vi "DAC.vi"() -> ()   [LabVIEW 2010]
uses:
  <vilib>/eio/EIONode/EIONode.xnode
  <vilib>/Platform/TimedLoop/XDataNode/wakeup.ctl
  <vilib>/Platform/TimedLoop/XDataNode/XDNodeRunTimeDep.lvlib
  <vilib>/Platform/TimedLoop/XDataNode/nitl_modes.ctl
  <vilib>/Platform/TimedLoop/XDataNode/timing_clust.ctl
  <vilib>/Platform/TimedLoop/XDataNode/XDataNode.xnode
panel:
  in  "setBufferGainV_DD":bool
  in  "setLDACMode":bool
  in  "dataAndControlResetButton":bool
  in  "stop":bool
  in  "V_DD":enum16{"as reference", "not as reference"}(ring)
  in  "Gain":enum16{"Range 0...V_ref", "Range 0...2V_ref"}(ring)
  in  "Buffer mode":enum16{"unbuffered", "buffered"}(ring)
  out "loop counter":i32
  out "write counter":i32
  out "current bit":bool
  out "U16 data word":bool[](array[boolean])
  in  "dataResetButton":bool
  in  "Channel":u8 max=7 step=1
  in  "Voltage":u16 max=4095
  in  "startButton":bool
  in  "LDAC mode":T1(ring)
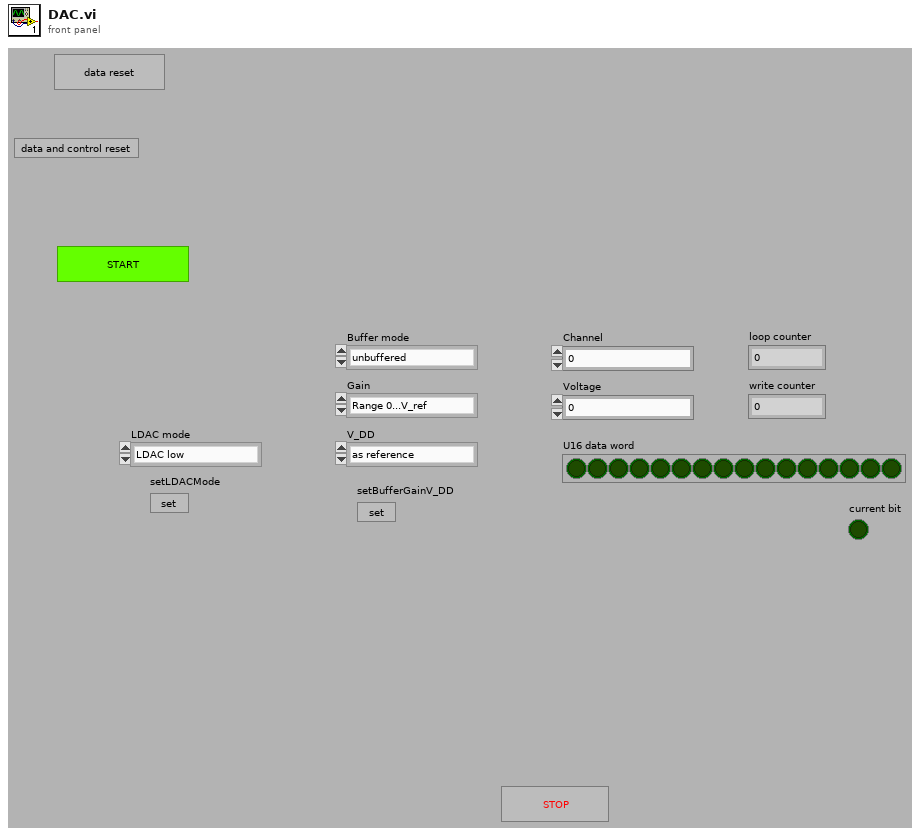
[diagram p1: front panel]
types:
  T1 = enum16{"LDAC low", "LDAC high", "LDAC single update"}
  T2 = typedef "XDNodeRunTimeDep.lvlib/timing_clust.ctl" = cluster{"Expected End [f-1]":u64, "Actual End [f-1]":u64, "Finished Late? [f-1]":bool, "Expected End [i-1]":u64, "Actual End [i-1]":u64, "Finished Late? [i-1]":bool, "Expected Start [i]":u64, "Actual Start [i]":u64, "Expected Start [f]":u64, "Actual Start [f]":u64, "Source Name":string, "Structure Name":string, "Period":i64, "Deadline":i64, "Offset":i64, "Start":i64, "Priority":i32, "Timeout":i32, "Mode":T3, "Wakeup Reason":T4, "Error":errorcluster, "Source Type":string, "Secondary Source Type":string, "Global End Time":u64, "Global Start Time":u64, "Frame Duration":u64, "Iteration Duration":u64, "Assigned CPU":i32, "I/O Scan Engine Mode":u32}
  T3 = typedef "XDNodeRunTimeDep.lvlib/nitl_modes.ctl" = enum32{"No Change", "Process missed periods, maintain original phase", "Discard missed periods, maintain original phase", "Process missed periods, ignore original phase", "Discard missed periods, ignore original phase"}
  T4 = typedef "XDNodeRunTimeDep.lvlib/wakeup.ctl" = enum32{"Normal", "Aborted", "Asynchronous wakeup", "Timing source error", "Timed loop error", "Timeout"}
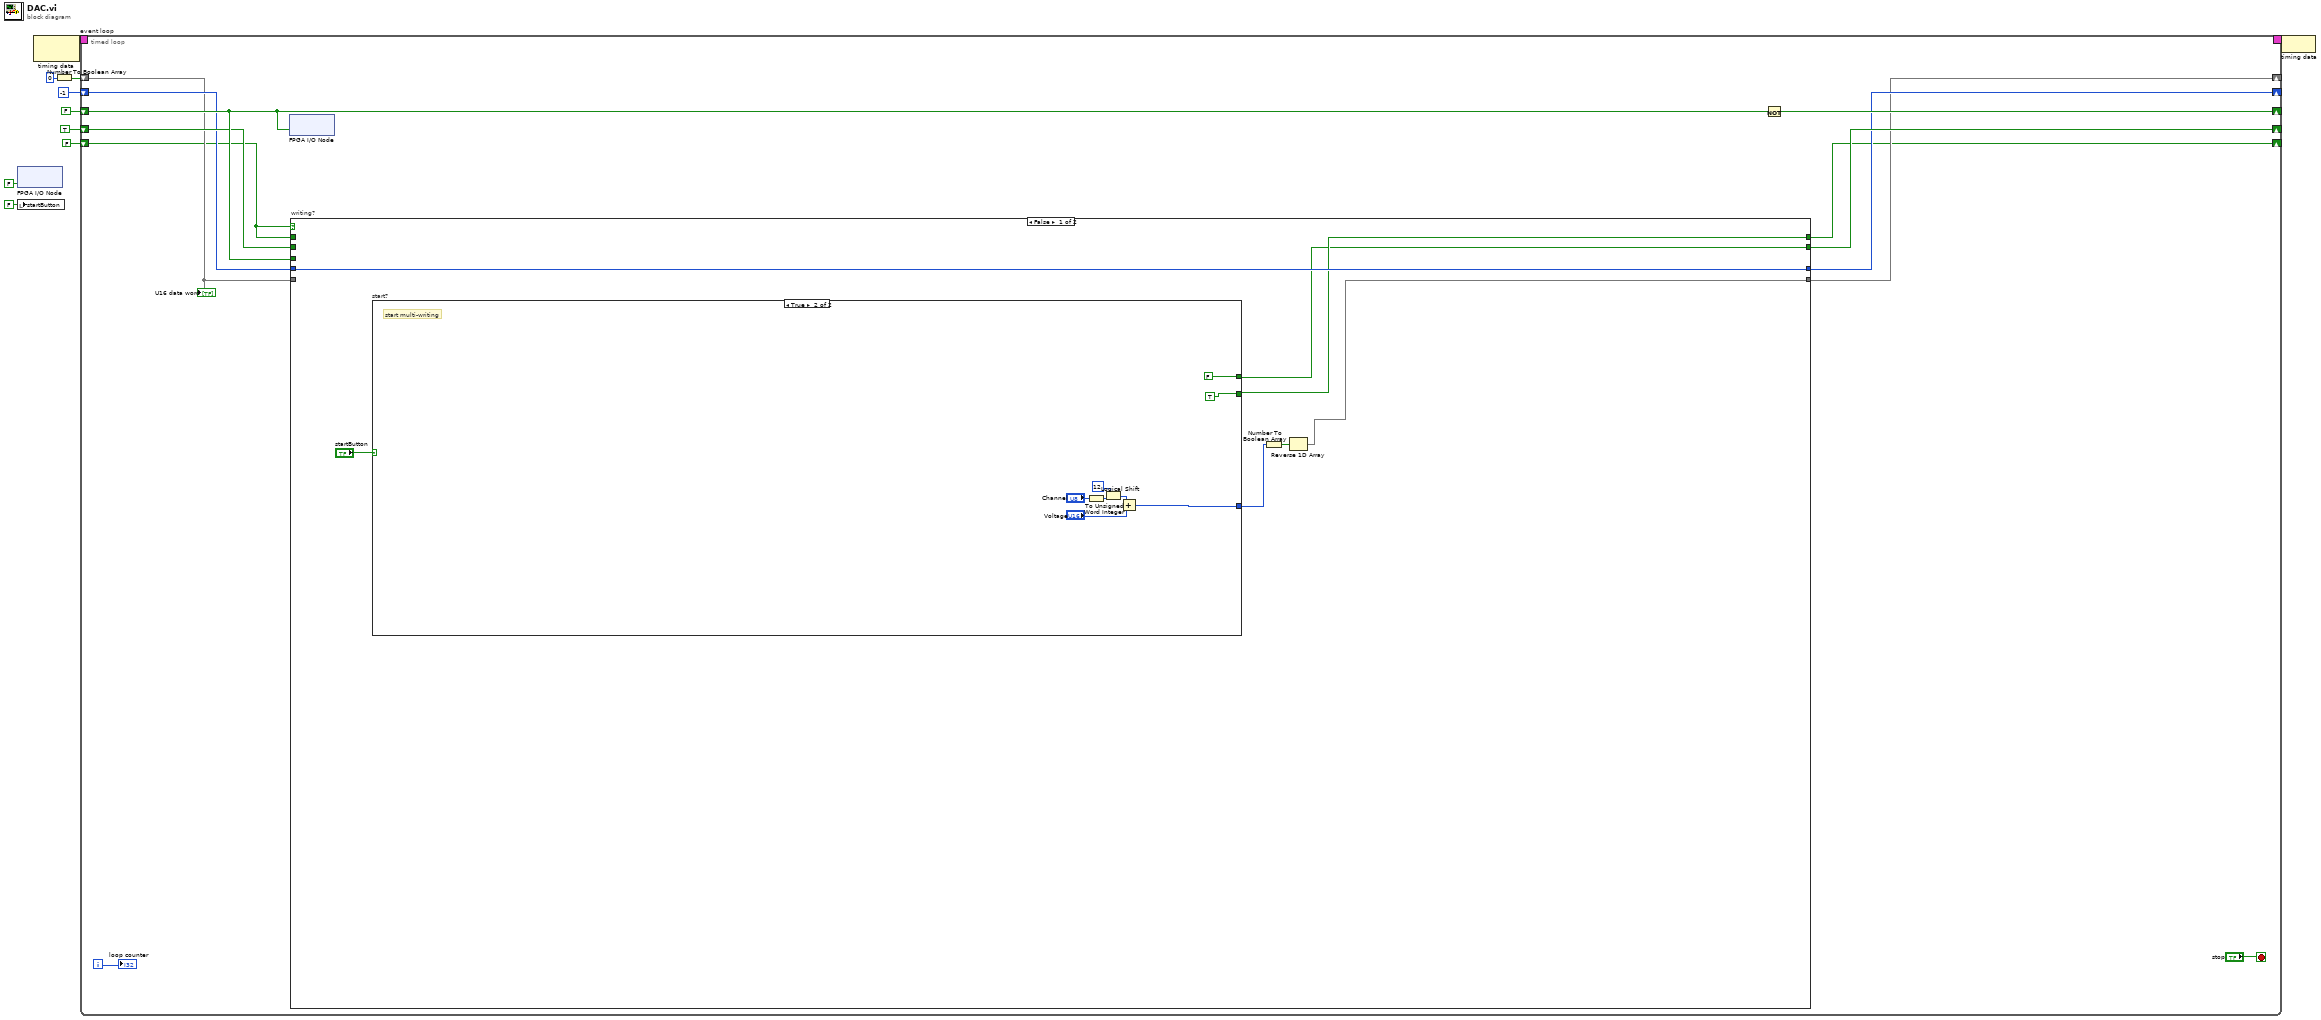
[diagram p0: block diagram]
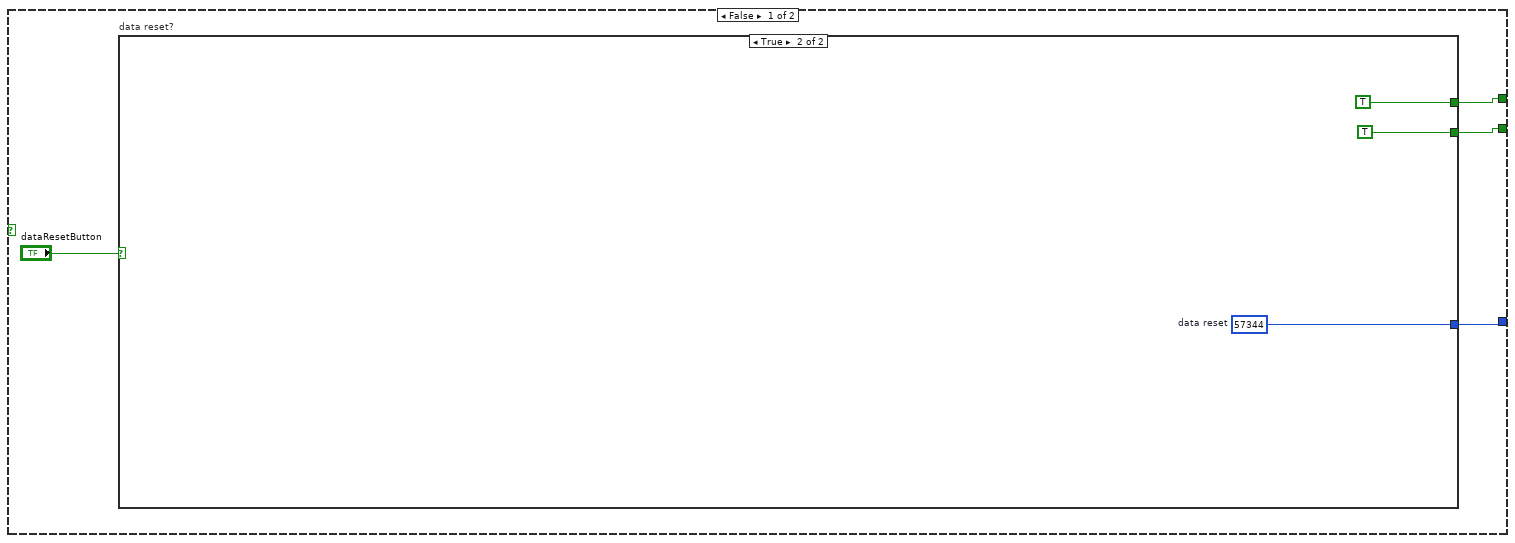
[diagram p2: hidden frame]
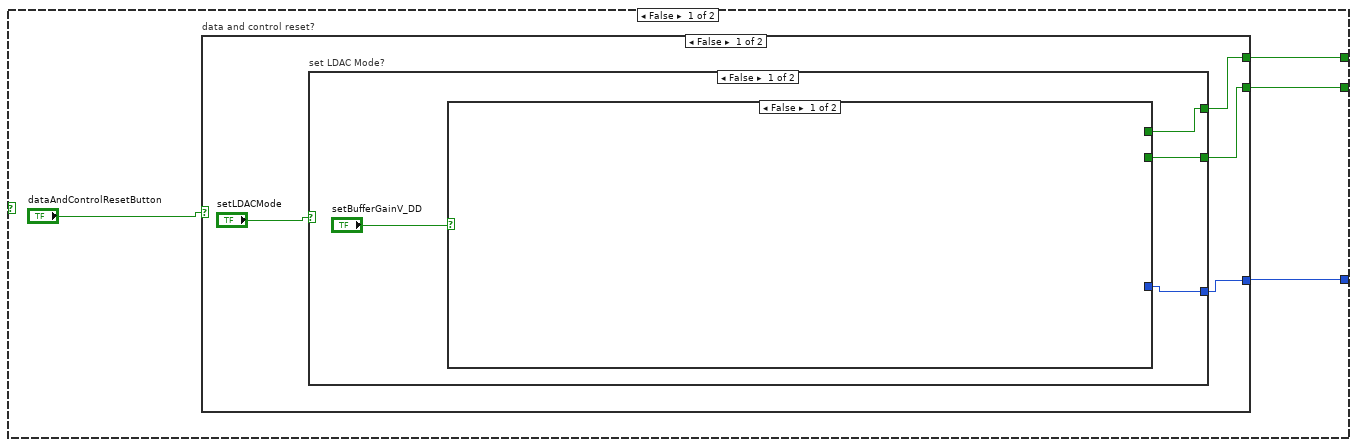
[diagram p3: hidden frame]
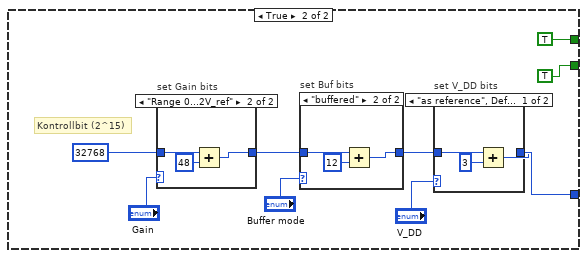
[diagram p4: hidden frame]
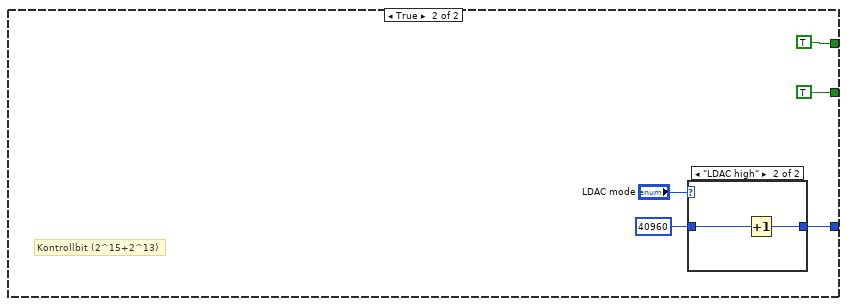
[diagram p8: hidden frame]
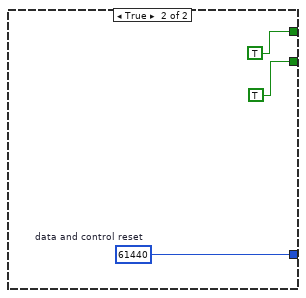
[diagram p10: hidden frame]
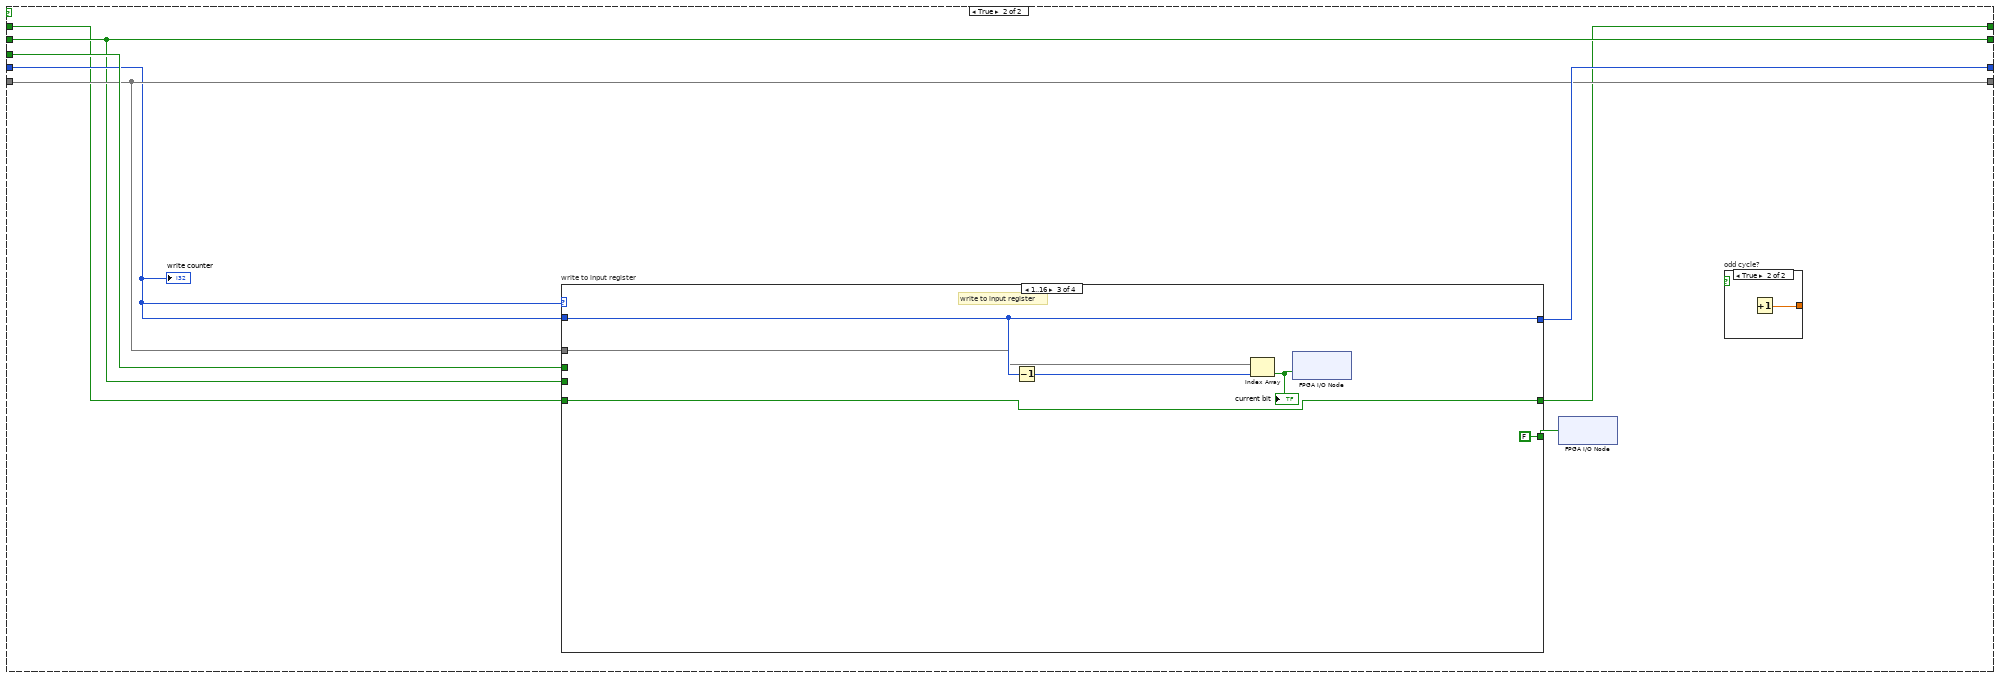
[diagram p11: hidden frame]
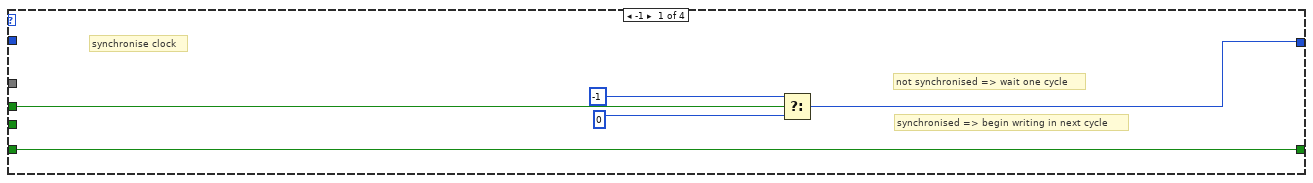
[diagram p12: hidden frame]
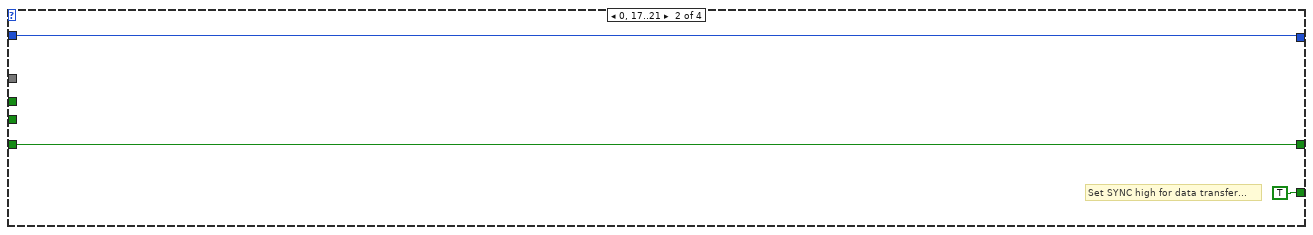
[diagram p13: hidden frame]
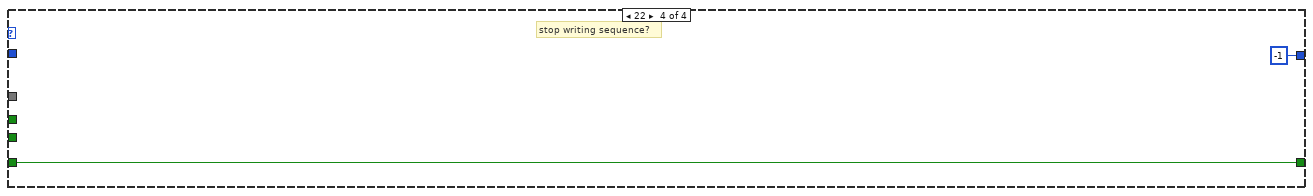
[diagram p14: hidden frame]
diagram:
  n1 = xnode "FPGA I/O Node"("LDAC"=FALSE) -> ()  [unwired: 1 in, 1 out]
  n2 = local write "startButton"(FALSE ("startButton")) -> ()
  n3 = node-c288() -> (w10:T2)  [unwired: 1 in]
  n4 = Number To Boolean Array(number=u16 0) -> (Boolean array=w4:bool[])
  n5 = timed-loop "event loop" {
    shift-right: [w17] -> _
    shift-left: TRUE -> [w18]
    shift-right: [w14] -> _
    shift-left: w4 -> [w13]
    timing: w10 -> [_]
    timing-out: [_] -> w9
    shift-right: [w15] -> _
    shift-left: -1 ("f") -> [w16]
    shift-right: [w21] -> _
    shift-left: FALSE -> [w20]
    shift-right: [w11] -> _
    shift-left: FALSE -> [w12]
    i -> [w22]
    stop <- "stop" stop-if-true
    n6 = xnode "FPGA I/O Node"("SCLK"=w20) -> ()  [unwired: 1 in, 1 out]
    n7 = case "writing?" shown="False" w12 {
      tunnel: w18 -> [_ w91]
      tunnel: w20 -> [_ w95]
      tunnel: w16 -> [w29 w92]
      tunnel: w13 -> [_ w93]
      tunnel: [w26 w91] -> w17
      tunnel: [w29 w94] -> w15
      tunnel: [w24 w93] -> w14
      tunnel: w12 -> [_ w90]
      tunnel: [w27 w89] -> w11
      frame False {
        n8 = case "start?" shown="True" "startButton" {
          tunnel: [w32 TRUE] -> w27
          tunnel: [w31 FALSE] -> w26
          tunnel: [w30 w81] -> w23
          frame False {
            n9 = case "data reset?" shown="True" "dataResetButton" {
              tunnel: [w35 TRUE] -> w32
              tunnel: [w36 TRUE] -> w31
              tunnel: [w34 w78] -> w30
              frame False {
                n10 = case "data and control reset?" shown="False" "dataAndControlResetButton" {
                  tunnel: [w39 TRUE] -> w36
                  tunnel: [w38 TRUE] -> w35
                  tunnel: [w40 w75] -> w34
                  frame False {
                    n11 = case "set LDAC Mode?" shown="False" "setLDACMode" {
                      tunnel: [w44 w69] -> w40
                      tunnel: [w43 TRUE] -> w39
                      tunnel: [w42 TRUE] -> w38
                      frame False {
                        n12 = case shown="False" "setBufferGainV_DD" {
                          tunnel: [_ w48] -> w44
                          tunnel: [_ TRUE] -> w43
                          tunnel: [_ TRUE] -> w42
                          frame False {
                          }
                          frame True {
                            # "Kontrollbit (2^15)"
                            n13 = case "set Gain bits" shown="\"Range 0...2V_ref\"" "Gain" {
                              tunnel: u16 32768 -> [w63 w66]
                              tunnel: [w63 w65] -> w52
                              frame "Range 0...V_ref", Default {
                              }
                              frame "Range 0...2V_ref" {
                                n14 = Add(x=w66, y=u16 48) -> (x+y=w65:u16)
                              }
                            }
                            n15 = case "set Buf bits" shown="\"buffered\"" "Buffer mode" {
                              tunnel: w52 -> [w59 w62]
                              tunnel: [w59 w61] -> w51
                              frame "unbuffered", Default {
                              }
                              frame "buffered" {
                                n16 = Add(x=w62, y=u16 12) -> (x+y=w61:u16)
                              }
                            }
                            n17 = case "set V_DD bits" shown="\"as reference\", Default" "V_DD" {
                              tunnel: w51 -> [w57 w58]
                              tunnel: [w56 w58] -> w48
                              frame "as reference", Default {
                                n18 = Add(x=w57, y=u16 3) -> (x+y=w56:u16)
                              }
                              frame "not as reference" {
                              }
                            }
                          }
                        }
                      }
                      frame True {
                        # "Kontrollbit (2^15+2^13)"
                        n19 = case shown="\"LDAC high\"" "LDAC mode" {
                          tunnel: u16 40960 -> [w72 w74]
                          tunnel: [w72 w73] -> w69
                          frame "LDAC low", Default {
                          }
                          frame "LDAC high" {
                            n20 = Increment(x=w74) -> (x+1=w73:u16)
                          }
                        }
                      }
                    }
                  }
                  frame True {
                    w75 = u16 61440  # data and control reset
                  }
                }
              }
              frame True {
                w78 = u16 57344  # data reset
              }
            }
          }
          frame True {
            # "start multi-writing"
            n21 = To Unsigned Word Integer(number="Channel") -> (unsigned 16bit integer=w86:u16)
            n22 = Logical Shift(y=i16 12, x=w86) -> (x << y=w87:u16)
            n23 = Add(x=w87, y="Voltage") -> (x+y=w81:u16)
          }
        }
        n24 = Number To Boolean Array(number=w23) -> (Boolean array=w25:bool[])
        n25 = Reverse 1D Array(array=w25) -> (reversed array=w24:bool[])
      }
      frame True {
        n26 = case "write to input register" shown="1..16" w92 {
          tunnel: [_ TRUE ("SYNC") FALSE ("SYNC") _] -> w96
          tunnel: w95 -> [w100 _ _ _]
          tunnel: w92 -> [_ w103 w109 _]
          tunnel: [w98 w103 w109 -1 ("f")] -> w94
          tunnel: w93 -> [_ _ w106 _]
          tunnel: w91 -> [_ _ _ _]
          tunnel: w90 -> [w97 w102 w105 w111]
          tunnel: [w97 w102 w105 w111] -> w89
          frame -1 {
            # "synchronise clock"
            # "not synchronised => wait one cycle"
            # "synchronised => begin writing in next cycle"
            n27 = Select(t=-1, s=w100, f=0) -> (s? t:f=w98:i32)
          }
          frame 0, 17..21 {
            # "Set SYNC high for data transfer..."
          }
          frame 1..16 {
            # "write to input register"
            n28 = Decrement(x=w109) -> (x-1=w108:i32)
            n29 = Index Array(array=w106, index=w108) -> (element=w107:bool)
            "current bit" <- w107
            n30 = xnode "FPGA I/O Node"("DIN"=w107) -> ()  [unwired: 1 in, 1 out]
          }
          frame 22 {
            # "stop writing sequence?"
          }
        }
        n31 = xnode "FPGA I/O Node"("SYNC"=w96) -> ()  [unwired: 1 in, 1 out]
        n32 = case "odd cycle?" shown="True" {
          selector: _ -> [_ _]
          tunnel: [_ w113] -> _
          frame False {
          }
          frame True {
            n33 = Increment() -> (x+1=w113:dbl)  [unwired: 1 in]
          }
        }
        "write counter" <- w92
      }
    }
    n34 = Not(x=w20) -> (.not. x?=w21:bool)
    "loop counter" <- w22
    "U16 data word" <- w13
  }
  n35 = node-c288(w9) -> ()
